vi "TOML sections.vi"() -> ()   [LabVIEW 2020]
doc: "This example VI demonstrates how to use the TOML library"
uses:
  lib/TOML Value.ctl
  3dd03dea-ebb6-4d13-ba4c-6119dc4e11fd.vi
  lib/TOML to LabVIEW.vi
  lib/LabVIEW to TOML.vi
  lib/TOML.lvlib
panel:
  in  "array_of_tables":T1(array[cluster])
  out "edit section error":errorcluster
  out "error":errorcluster caption="LV to TOML error"
  out "TOML to LV error":errorcluster
  in  "support-path":cluster{"file-windows":path, "file-linux":path}
  in  "clients":cluster{"hosts":string[], "data":string[][]}
  in  "database":T2
  in  "Fail":bool
  out "toml":string caption="new TOML String"
  in  "original TOML String":string
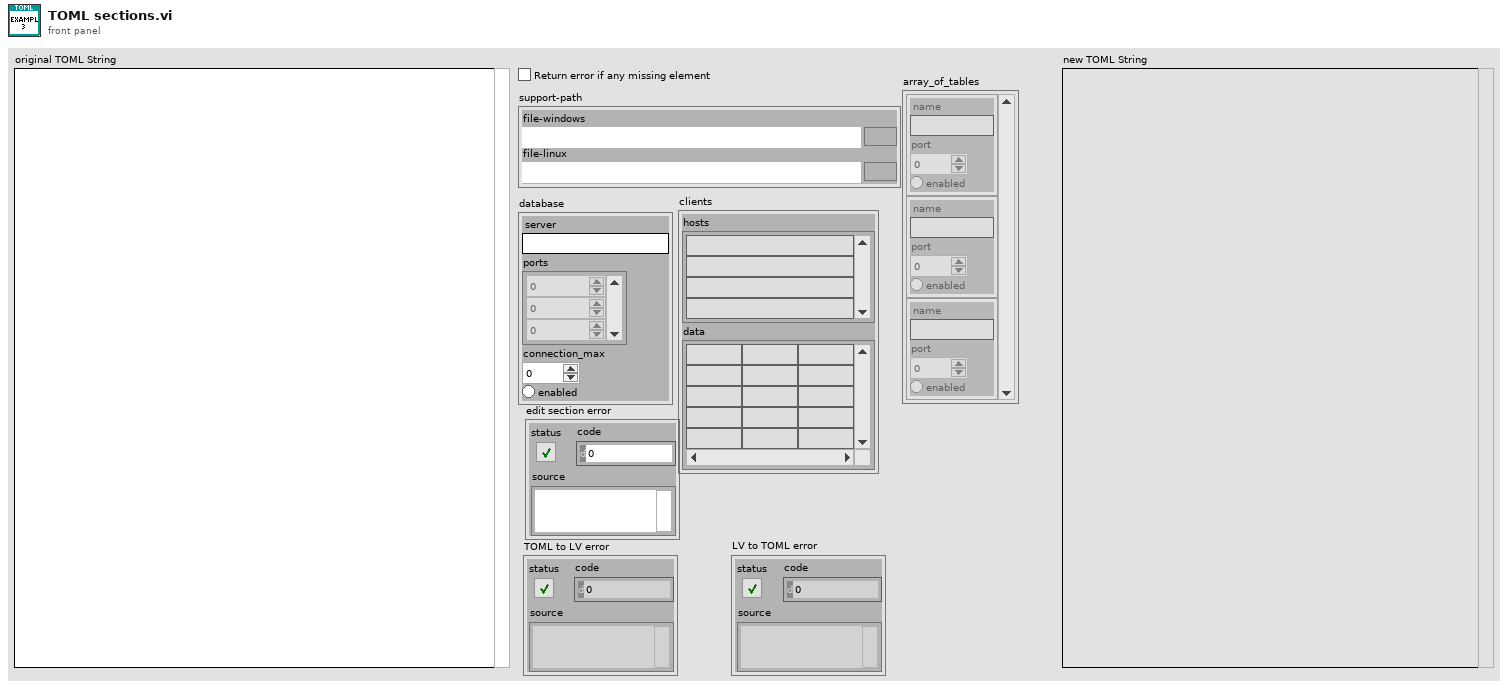
[diagram p1: front panel]
types:
  T1 = cluster{"name":string, "port":u16, "enabled":bool}[]
  T2 = cluster{"server":string, "ports":u16[], "connection_max":dbl, "enabled":bool}
  T3 = typedef "TOML.lvlib/TOML Value.ctl" = cluster{"type":enum16{"Table", "Array", "String", "Integer", "Float", "Boolean", "Offset Date-Time", "Local Date-Time", "Local Date", "Local Time", "Path"}, "value":variant}
  T4 = cluster{"database":cluster{"server":string, "ports":u16[], "connection_max":dbl, "enabled":bool}, "clients":cluster{"hosts":string[], "data":string[][]}, "support-path":cluster{"file-windows":path, "file-linux":path}, "array_of_tables":cluster{"name":string, "port":u16, "enabled":bool}[]}
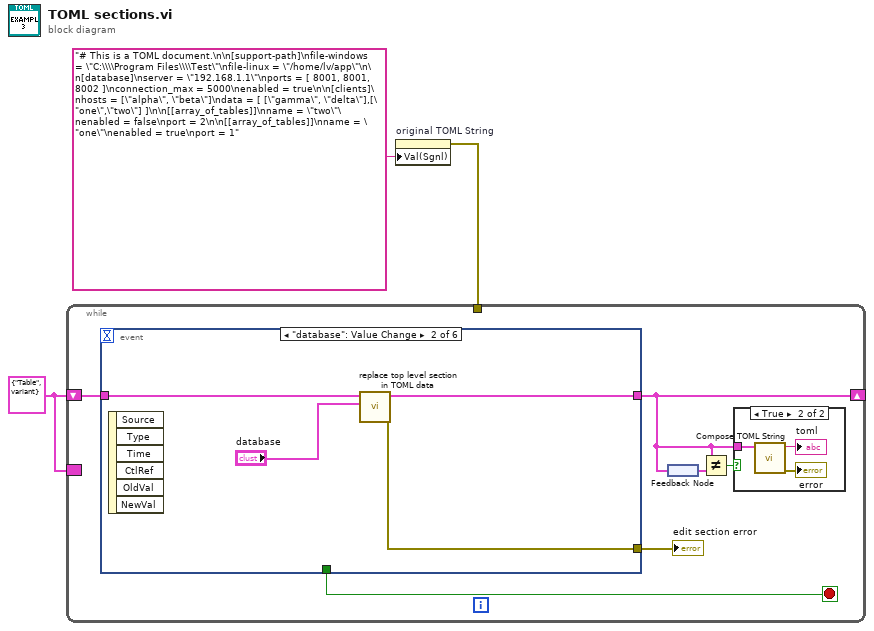
[diagram p0: block diagram]
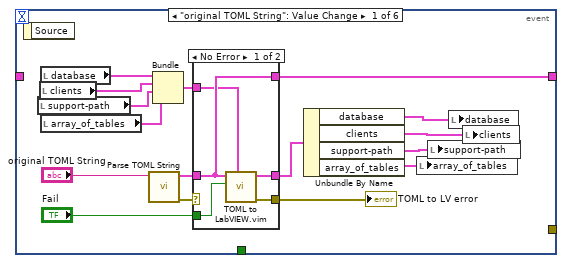
[diagram p3: hidden frame]
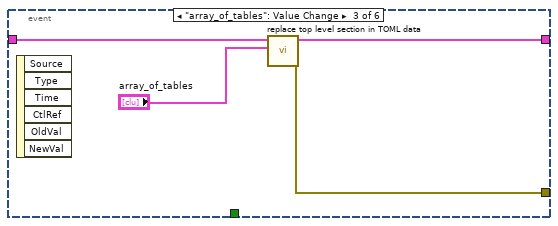
[diagram p5: hidden frame]
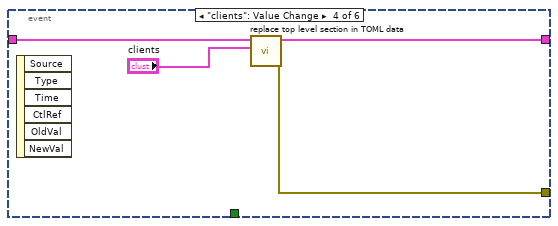
[diagram p6: hidden frame]
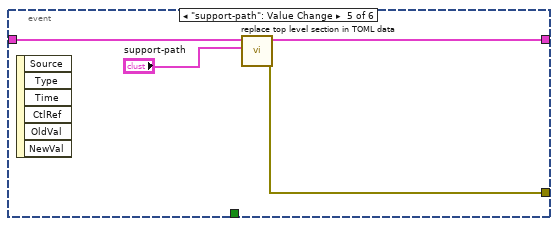
[diagram p7: hidden frame]
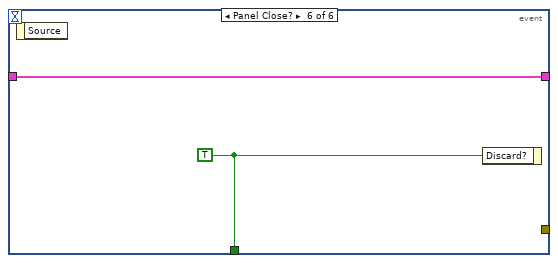
[diagram p8: hidden frame]
diagram:
  w1 = T3 {"type"=enum."Table", "value"=variant} ("Value")
  n1 = property on="original TOML String" class="Str"("Val(Sgnl)"="# This is a TOML document.\n\n[support-path]\nfile-windows = \"C:\\\\Program Files\\\\Test\"\nfile-linux = \"/home/lv/app\"\n\n[database]\nserver = \"192.168.1.1\"\nports = [ 8001, 8001, 8002 ]\nconnection_max = 5000\nenabled = true\n\n[clients]\nhosts = [\"alpha\", \"beta\"]\ndata = [ [\"gamma\", \"delta\"],[\"one\",\"two\"] ]\n\n[[array_of_tables]]\nname = \"two\"\nenabled = false\nport = 2\n\n[[array_of_tables]]\nname = \"one\"\nenabled = true\nport = 1" ("TOML String")) -> (error out=w2:errorcluster)  [unwired: 2 in, 1 out]
  n2 = while {
    tunnel: w2 -> [_]
    shift-right: [w6] -> _
    shift-left: w1 -> [w7]
    border: w1 -> [_]
    stop <- w9 stop-if-true
    n3 = event shown="[1] \"database\": Value Change" {
      selector: _ -> [_ _ _ _ _ _]
      dyn-events: _ -> [_ _ _ _ _ _]
      timeout: _ -> [_ _ _ _ _ _]
      tunnel: [_ _ _ _ _ w52] -> w9
      tunnel: [w14 w36 w41 w45 w49 w51] -> w6
      tunnel: w7 -> [_ w37 w42 w46 w50 w51]
      tunnel: [_ w35 w40 w43 w48 _] -> w4
      event "original TOML String": Value Change {
        n4 = event-data() -> ()  [unwired: 1 in, 1 out]
        n5 = local read "support-path"() -> (w18:cluster{"file-windows":path, "file-linux":path})
        n6 = local read "clients"() -> (w19:cluster{"hosts":string[], "data":string[][]})
        n7 = local read "database"() -> (w20:T2)
        n8 = local read "array_of_tables"() -> (w16:T1)
        n9 = call "Parse TOML String.vi"("String"="original TOML String") -> ("error out"=w28:errorcluster, "Value"=w27:T3)  [unwired: 9 in]
        n10 = Bundle("database"=w20, "clients"=w19, "support-path"=w18, "array_of_tables"=w16) -> (w17:T4)  [unwired: 1 in]
        n11 = case shown="No Error" w28 {
          selector: w28 -> [_ w34]
          tunnel: w27 -> [w30 _]
          tunnel: [w33 _] -> w22
          tunnel: "Fail" -> [w32 _]
          tunnel: [w31 w34] -> w23
          tunnel: [w30 _] -> w14
          tunnel: w17 -> [w29 _]
          frame No Error {
            n12 = call "TOML to LabVIEW.vim"("datatype"=w29, "Error if missing element"=w32, "Value"=w30) -> ("error out"=w31:errorcluster, "LV Data"=w33:T4)  [unwired: 6 in, 1 out]
          }
          frame Error {
          }
        }
        "TOML to LV error" <- w23
        n13 = Unbundle By Name(w22) -> ("database"=w13:T2, "clients"=w25:cluster{"hosts":string[], "data":string[][]}, "support-path"=w24:cluster{"file-windows":path, "file-linux":path}, "array_of_tables"=w15:T1)
        n14 = local write "array_of_tables"(w15) -> ()
        n15 = local write "support-path"(w24) -> ()
        n16 = local write "database"(w13) -> ()
        n17 = local write "clients"(w25) -> ()
      }
      event "database": Value Change {
        n18 = event-data() -> ()  [unwired: 1 in, 6 out]
        n19 = call "replace top level section in TOML data.vi"("Section data"="database", "Value in"=w37) -> ("error out"=w35:errorcluster, "Value out"=w36:T3)  [unwired: 8 in]
      }
      event "array_of_tables": Value Change {
        n20 = event-data() -> ()  [unwired: 1 in, 6 out]
        n21 = call "replace top level section in TOML data.vi"("Section data"="array_of_tables", "Value in"=w42) -> ("error out"=w40:errorcluster, "Value out"=w41:T3)  [unwired: 8 in]
      }
      event "clients": Value Change {
        n22 = event-data() -> ()  [unwired: 1 in, 6 out]
        n23 = call "replace top level section in TOML data.vi"("Section data"="clients", "Value in"=w46) -> ("error out"=w43:errorcluster, "Value out"=w45:T3)  [unwired: 8 in]
      }
      event "support-path": Value Change {
        n24 = event-data() -> ()  [unwired: 1 in, 6 out]
        n25 = call "replace top level section in TOML data.vi"("Section data"="support-path", "Value in"=w50) -> ("error out"=w48:errorcluster, "Value out"=w49:T3)  [unwired: 8 in]
      }
      event Panel Close? {
        w52 = TRUE
        n26 = event-data() -> ()  [unwired: 1 in, 1 out]
        n27 = event-data("Discard?"=w52) -> ()  [unwired: 1 in, 1 out]
      }
    }
    "edit section error" <- w4
    n28 = feedback #1() -> (w5:T3)
    n29 = feedback-in #1(w6) -> ()
    n30 = Not Equal?(x=w6, y=w5) -> (x != y?=w8:bool)
    n31 = case shown="True" w8 {
      tunnel: w6 -> [_ w10]
      frame False {
      }
      frame True {
        n32 = call "Compose TOML String.vi"("Value"=w10) -> ("error out"=→"error":errorcluster, "String"=→"toml":string)  [unwired: 9 in]
      }
    }
  }
